vi "Log.vi"(8 "error in (no error)":errorcluster, 10 "message":string, 11 "id":i32) -> (0 "error out":errorcluster)   [LabVIEW 2020, in "MCP Server.lvlib"]
uses:
  MCP Server.lvlib
  onLog.ctl
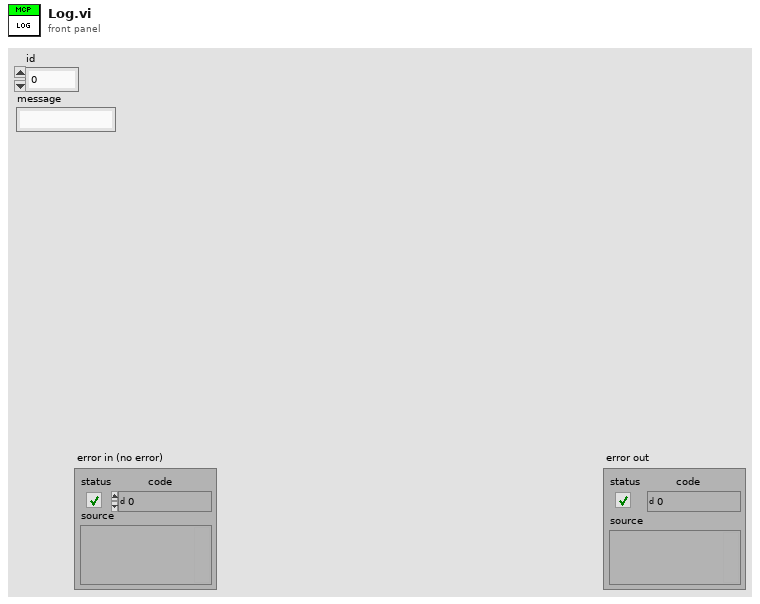
[diagram p1: front panel]
types:
  T1 = typedef "MCP Server.lvlib/onLog.ctl" = cluster{"message":string}
  T2 = typedef "MCP Server.lvlib/Server Data.ctl" = cluster{"Name":string, "Description":string, "Tools":T3[], "Parameters":string[][], "Logging Info":T6, "User Events":T7, "Prompts":T8[], "resources":T10[], "HTTP Server":refnum<class "Server.lvclass">}
  T3 = typedef "MCP Server.lvlib/Tool Data.ctl" = cluster{"Name":string, "Description":string, "Ignored":string[], "inputs":T4[], "outputs":T5[], "VI Refnum":refnum<vi>}
  T4 = typedef "MCP Server.lvlib/Input Parameter.ctl" = cluster{"name":string, "type":string, "description":string, "required":bool, "raw name":string}
  T5 = typedef "MCP Server.lvlib/Output Parameter.ctl" = cluster{"name":string, "description":string, "type":string, "raw name":string}
  T6 = typedef "MCP Server.lvlib/Logging.ctl" = cluster{"Log":string[], "Max Length":i32}
  T7 = typedef "MCP Server.lvlib/User Events.ctl" = cluster{"onError":refnum<user-event>, "onRpc":refnum<user-event>}
  T8 = typedef "MCP Server.lvlib/Prompt Data.ctl" = cluster{"name":string, "description":string, "arguments":T9[], "return terminal name":string, "results description":string, "VI Refnum":refnum<vi>}
  T9 = typedef "MCP Server.lvlib/Prompt Argument.ctl" = cluster{"name":string, "description":string, "required":bool, "raw_name":string}
  T10 = typedef "MCP Server.lvlib/resource data.ctl" = cluster{"uri":string, "name":string, "description":string, "mimeType":string, "file path":path}
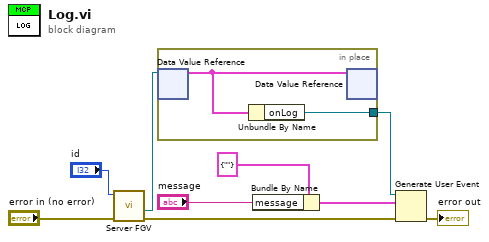
[diagram p0: block diagram]
diagram:
  n1 = call "Server FGV.vi"("error in"="error in (no error)", "id"="id") -> ("error out"=w8:errorcluster, "server reference"=w5:refnum<data-value>)  [unwired: 5 in, 3 out]
  n2 = in-place {
    in-place-border: [w10] -> w4
    n3 = in-place-dvr #1(w5) -> (w11:T2)  [unwired: 1 out]
    n4 = Unbundle By Name(w11) -> ("onLog"=w10:refnum<user-event>)
    n5 = in-place-dvr #1(w11) -> ()  [unwired: 2 out]
  }
  n6 = Bundle By Name(cluster=T1 {"message"=""} ("event data"), "message"="message") -> (w2:T1)
  n7 = Generate User Event(user event=w4, event data cluster=w2, error in=w8) -> (error out=→"error out":errorcluster)  [unwired: 1 in, 1 out]
